vi "Calibration - Oxygen.vi"() -> ()   [LabVIEW 2016]
uses:
  calibration states.ctl
panel:
  out "Read indicator":bool
  out "Reading, mg/L":dbl
  in  "Calibrate2":bool
  out "Status":string
  in  "Cancel":bool
  in  "Calibrate1":bool
  # "ATLAS SCIENTIFIC\nOXYGEN SENSOR CALIBRATION"
  # "1. Calibrate in air:\n- Pull off the cap from the Dissolved Oxygen probe.\n- Let the Dissolved Oxygen probe sit, exposed to air (5 – 30 sec).\n- Calibrate using the command \"Calibrate in air\".\n- After calibration is complete, you should see readings ~9.09 – 9.1 mg/L\n\n2. Calibrate in solution (Only perform this calibration if you require accurate readings below 1.0 mg/L)\n- Stir probe in Zero D.O. calibration solution to remove trapped air (which could cause readings to go high).\n- Let the probe sit in Zero D.O. calibration solution untill readings stabilize (10 – 90 sec).\n- Calibrate using the command \"Calibrate in solution\"."
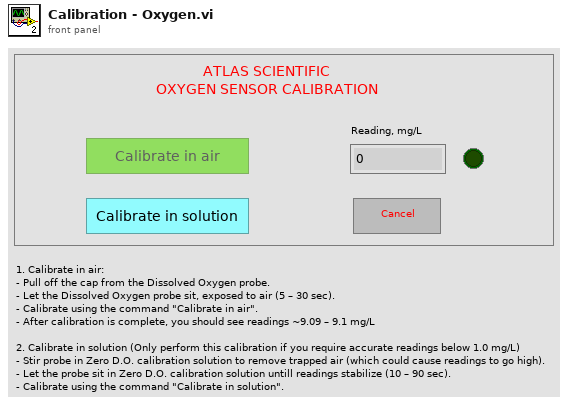
[diagram p1: front panel]
types:
  T1 = enum32{"Invalid", "Standard", "Closed", "Hidden", "Minimized", "Maximized"}
  T2 = typedef "Visa com cluster def (subVI).ctl" = cluster{"Sensor":string, "VISA resource name":refnum<visa-resource-name>, "error in/out":errorcluster, "bytes read":u32, "Com found ?":bool}
  T3 = typedef "calibration states.ctl" = string
  T4 = enum8{"Enabled", "Disabled", "Disabled and Grayed Out"}
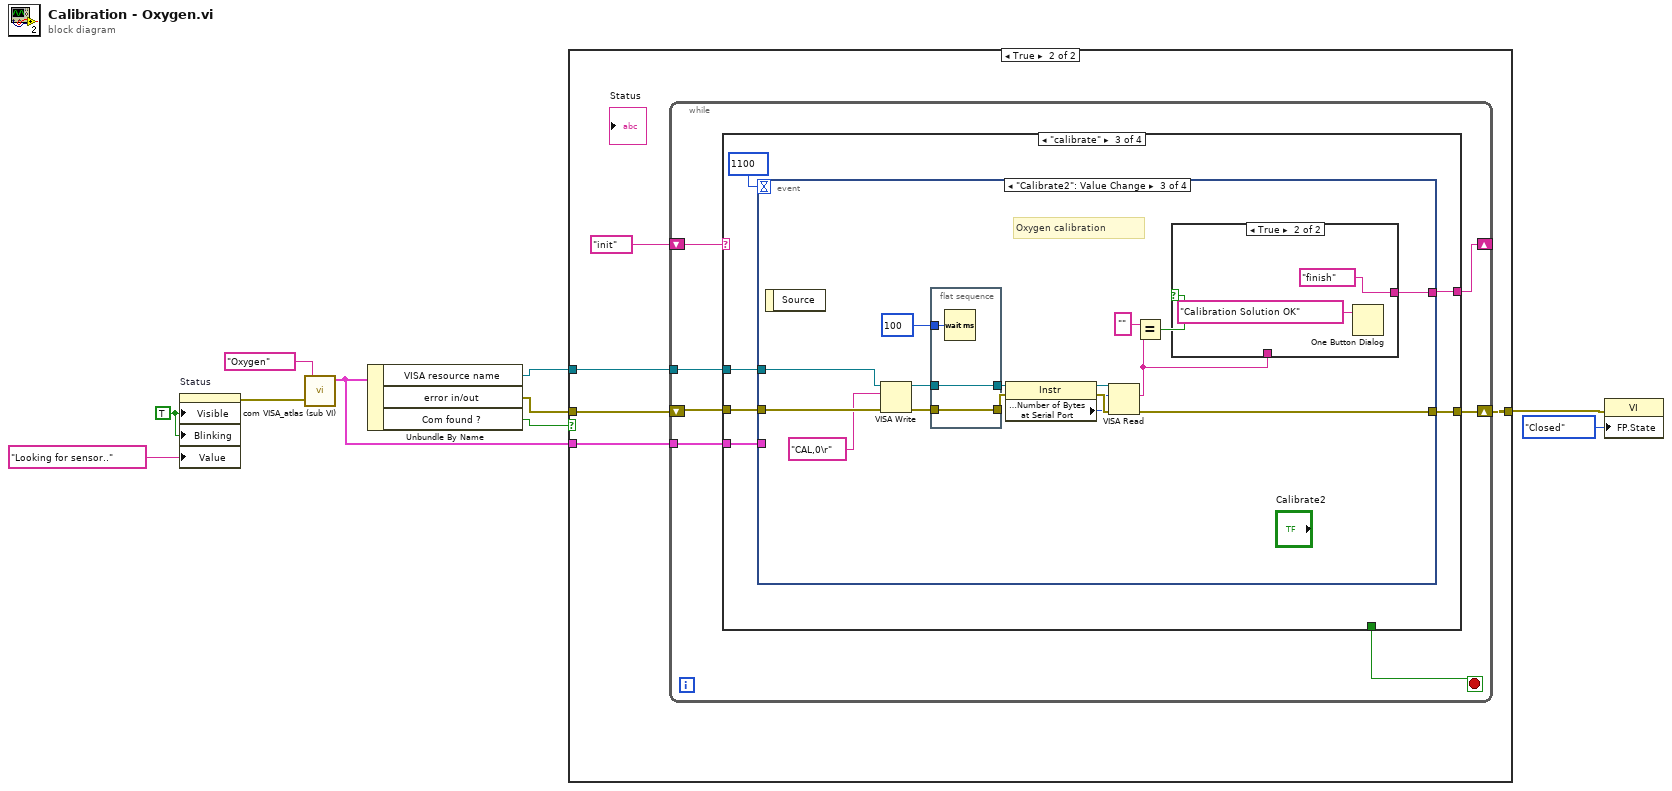
[diagram p0: block diagram]
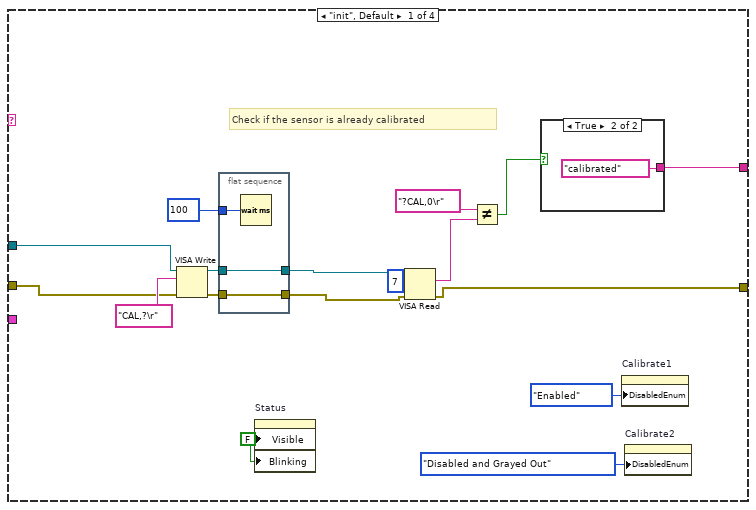
[diagram p3: hidden frame]
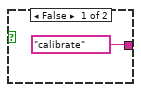
[diagram p4: hidden frame]
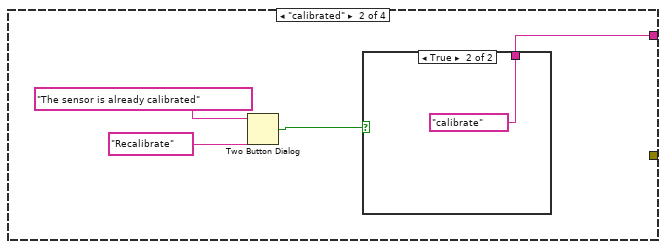
[diagram p5: hidden frame]
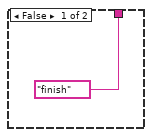
[diagram p6: hidden frame]
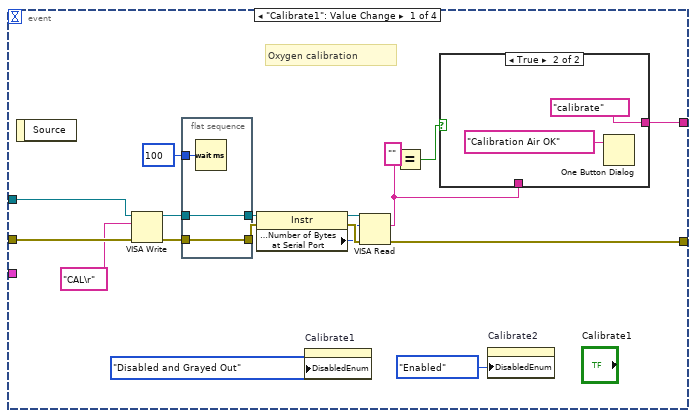
[diagram p7: hidden frame]
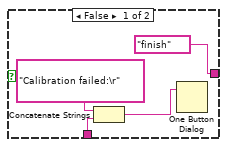
[diagram p8: hidden frame]
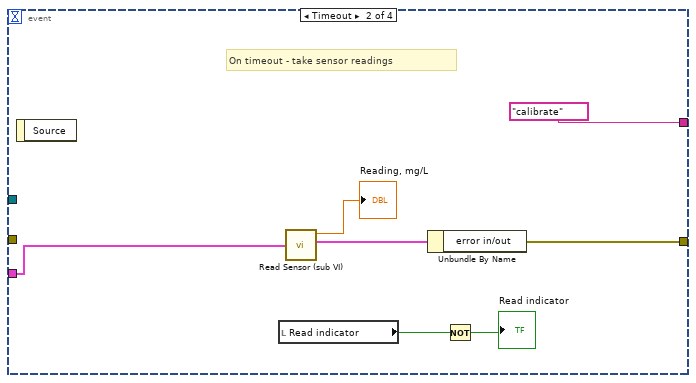
[diagram p9: hidden frame]
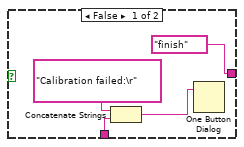
[diagram p10: hidden frame]
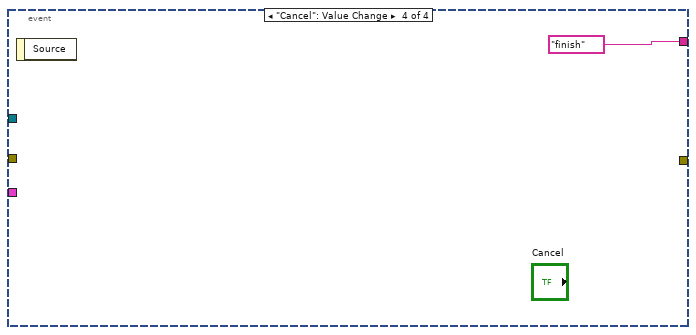
[diagram p11: hidden frame]
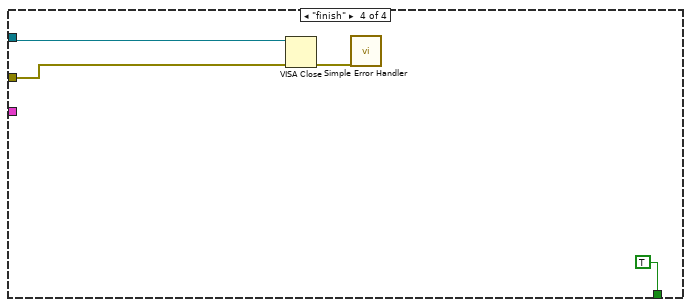
[diagram p12: hidden frame]
diagram:
  w10 = TRUE ("Visible")
  n1 = property on="Status" class="Str"("Visible"=w10, "Blinking"=w10, "Value"="Looking for sensor.." ("Status")) -> (error out=w6:errorcluster)  [unwired: 2 in, 1 out]
  n2 = call "com VISA_atlas (sub VI).vi"("Sensor"="Oxygen", "entrée d'erreur (pas d'erreur)"=w6) -> ("Output cluster"=w5:T2)  [unwired: 2 in, 1 out]
  n3 = Unbundle By Name(w5) -> ("VISA resource name"=w8:refnum<visa-resource-name>, "error in/out"=w7:errorcluster, "Com found ?"=w1:bool)
  n4 = case shown="True" w1 {
    tunnel: w8 -> [_ w14]
    tunnel: w7 -> [_ w13]
    tunnel: w5 -> [_ w12]
    tunnel: [_ w11] -> w2
    frame False {
    }
    frame True {
      n5 = while {
        tunnel: w14 -> [w21]
        shift-right: [w20] -> _
        shift-left: T3 "init" ("State Calibr") -> [w22]
        shift-right: [w17] -> w11
        shift-left: w13 -> [w18]
        tunnel: w12 -> [w16]
        stop <- w19 stop-if-true
        n6 = case shown="\"calibrate\"" w22 {
          tunnel: w21 -> [w31 _ w56 w118]
          tunnel: [w29 w45 w55 _] -> w20
          tunnel: [_ _ _ TRUE] -> w19
          tunnel: w18 -> [w27 _ w54 w117]
          tunnel: [w26 _ w53 _] -> w17
          tunnel: w16 -> [_ _ w51 _]
          frame "init", Default {
            w25 = FALSE ("Visible")
            # "Check if the sensor is already calibrated"
            n7 = VISA Write(VISA resource name=w31, write buffer="CAL,?\r", error in (no error)=w27) -> (VISA resource name out=w33:refnum<visa-resource-name>, error out=w32:errorcluster)  [unwired: 1 out]
            n8 = flat-sequence {
              tunnel: w32 -> [w43]
              tunnel: [w43] -> w37
              tunnel: w33 -> [w42]
              tunnel: [w42] -> w39
              tunnel: u32 100 ("delay before read (ms)") -> [w44]
              frame #0 {
                n9 = Wait (ms)(milliseconds to wait=w44) -> ()  [unwired: 1 out]
              }
            }
            n10 = property on="Status" class="Str"("Visible"=w25, "Blinking"=w25) -> ()  [unwired: 2 in, 2 out]
            n11 = VISA Read(VISA resource name=w39, byte count=u32 7, error in (no error)=w37) -> (read buffer=w28:string, error out=w26:errorcluster)  [unwired: 2 out]
            n12 = Not Equal?(x="?CAL,0\r" ("Response 2"), y=w28) -> (x != y?=w30:bool)
            n13 = case shown="True" w30 {
              tunnel: [T3 "calibrate" ("State Calibr") T3 "calibrated" ("State Calibr")] -> w29
              frame False {
              }
              frame True {
              }
            }
            n14 = property on="Calibrate1" class="Bool"("DisabledEnum"=T4."Enabled" ("Disabled")) -> ()  [unwired: 2 in, 2 out]
            n15 = property on="Calibrate2" class="Bool"("DisabledEnum"=T4."Disabled and Grayed Out" ("Disabled")) -> ()  [unwired: 2 in, 2 out]
          }
          frame "calibrated" {
            n16 = Two Button Dialog(message="The sensor is already calibrated", 2:"Recalibrate" ("T button name (\"OK\")")) -> (T button?=w46:bool)  [unwired: 1 in]
            n17 = case shown="True" w46 {
              tunnel: [T3 "finish" ("State Calibr") T3 "calibrate" ("State Calibr")] -> w45
              frame False {
              }
              frame True {
              }
            }
          }
          frame "calibrate" {
            n18 = event shown="[2] \"Calibrate2\": Value Change" {
              selector: _ -> [_ _ _ _]
              dyn-events: _ -> [_ _ _ _]
              timeout: 1100 -> [_ _ _ _]
              tunnel: w56 -> [w70 _ w102 _]
              tunnel: [w64 T3 "calibrate" ("State Calibr") w96 T3 "finish" ("State Calibr")] -> w55
              tunnel: w54 -> [w61 _ w93 _]
              tunnel: [w60 w84 w92 _] -> w53
              tunnel: w51 -> [_ w86 _ _]
              event "Calibrate1": Value Change {
                # "Oxygen calibration"
                n19 = event-data() -> ()  [unwired: 1 in, 1 out]
                n20 = VISA Write(VISA resource name=w70, write buffer="CAL\r" ("format string"), error in (no error)=w61) -> (VISA resource name out=w73:refnum<visa-resource-name>, error out=w74:errorcluster)  [unwired: 1 out]
                n21 = flat-sequence {
                  tunnel: w74 -> [w76]
                  tunnel: [w76] -> w66
                  tunnel: w73 -> [w75]
                  tunnel: [w75] -> w65
                  tunnel: u32 100 ("delay before read (ms)") -> [w77]
                  frame #0 {
                    n22 = Wait (ms)(milliseconds to wait=w77) -> ()  [unwired: 1 out]
                  }
                }
                n23 = property class="Instr"(reference=w65, error in=w66) -> (reference out=w69:refnum<visa-resource-name>, error out=w68:errorcluster, "Serial Settings:Number of Bytes at Serial Port"=w67:u32)
                n24 = property on="Calibrate1" class="Bool"("DisabledEnum"=T4."Disabled and Grayed Out" ("Disabled")) -> ()  [unwired: 2 in, 2 out]
                n25 = VISA Read(VISA resource name=w69, byte count=w67, error in (no error)=w68) -> (read buffer=w62:string, error out=w60:errorcluster)  [unwired: 2 out]
                n26 = Equal?(x="" ("Response 2"), y=w62) -> (x = y?=w63:bool)
                n27 = case shown="True" w63 {
                  tunnel: [T3 "finish" ("State Calibr") T3 "calibrate" ("State Calibr")] -> w64
                  tunnel: w62 -> [w80 _]
                  frame False {
                    n28 = Concatenate Strings("Calibration failed:\r" ("message"), w80) -> (w78:string)
                    n29 = One Button Dialog(message=w78) -> ()  [unwired: 1 in, 1 out]
                  }
                  frame True {
                    n30 = One Button Dialog(message="Calibration Air OK") -> ()  [unwired: 1 in, 1 out]
                  }
                }
                n31 = property on="Calibrate2" class="Bool"("DisabledEnum"=T4."Enabled" ("Disabled")) -> ()  [unwired: 2 in, 2 out]
              }
              event Timeout {
                # "On timeout - take sensor readings"
                n32 = event-data() -> ()  [unwired: 1 in, 1 out]
                n33 = local read "Read indicator"() -> (w88:bool)
                n34 = call "Read Sensor (sub VI).vi"("Input cluster"=w86) -> ("Reading"=→"Reading, mg/L":dbl, "Output cluster"=w85:T2)  [unwired: 2 in]
                n35 = Unbundle By Name(w85) -> ("error in/out"=w84:errorcluster)
                n36 = Not(x=w88) -> (.not. x?=→"Read indicator":bool)
              }
              event "Calibrate2": Value Change {
                # "Oxygen calibration"
                n37 = event-data() -> ()  [unwired: 1 in, 1 out]
                n38 = VISA Write(VISA resource name=w102, write buffer="CAL,0\r" ("format string"), error in (no error)=w93) -> (VISA resource name out=w105:refnum<visa-resource-name>, error out=w106:errorcluster)  [unwired: 1 out]
                n39 = flat-sequence {
                  tunnel: w106 -> [w108]
                  tunnel: [w108] -> w98
                  tunnel: w105 -> [w107]
                  tunnel: [w107] -> w97
                  tunnel: u32 100 ("delay before read (ms)") -> [w109]
                  frame #0 {
                    n40 = Wait (ms)(milliseconds to wait=w109) -> ()  [unwired: 1 out]
                  }
                }
                n41 = property class="Instr"(reference=w97, error in=w98) -> (reference out=w101:refnum<visa-resource-name>, error out=w100:errorcluster, "Serial Settings:Number of Bytes at Serial Port"=w99:u32)
                n42 = VISA Read(VISA resource name=w101, byte count=w99, error in (no error)=w100) -> (read buffer=w94:string, error out=w92:errorcluster)  [unwired: 2 out]
                n43 = Equal?(x="" ("Response 2"), y=w94) -> (x = y?=w95:bool)
                n44 = case shown="True" w95 {
                  tunnel: [T3 "finish" ("State Calibr") T3 "finish" ("State Calibr")] -> w96
                  tunnel: w94 -> [w112 _]
                  frame False {
                    n45 = Concatenate Strings("Calibration failed:\r" ("message"), w112) -> (w110:string)
                    n46 = One Button Dialog(message=w110) -> ()  [unwired: 1 in, 1 out]
                  }
                  frame True {
                    n47 = One Button Dialog(message="Calibration Solution OK") -> ()  [unwired: 1 in, 1 out]
                  }
                }
              }
              event "Cancel": Value Change {
                n48 = event-data() -> ()  [unwired: 1 in, 1 out]
              }
            }
          }
          frame "finish" {
            n49 = VISA Close(VISA resource name=w118, error in (no error)=w117) -> (error out=w119:errorcluster)
            n50 = call <vilib>:"Simple Error Handler.vi"("error in (no error)"=w119) -> ()  [unwired: 1 in, 8 out]
          }
        }
      }
    }
  }
  n51 = property class="VI"(error in=w2, "FP.State"=T1."Closed" ("Front Panel Window:State")) -> ()  [unwired: 1 in, 2 out]
